vi "Over Awesome stuff.vi"() -> ()   [LabVIEW 2017]
uses:
  Gluing Procedure.lvclass
panel:
  out "Gluing Procedure out":refnum<class "Gluing Procedure.lvclass">
  in  "Gluing Procedure in":refnum<class "Gluing Procedure.lvclass">
  out "error out":errorcluster
  in  "error in":errorcluster
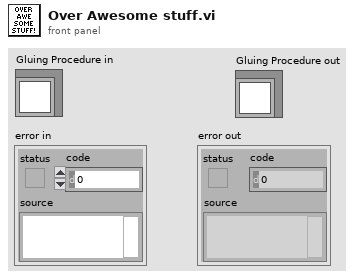
[diagram p1: front panel]
types:
  T1 = typedef "Configure.ctl" = cluster{"Has been run?":bool, "Active Paths":T2, "Glue Pathways":T3, "Chuck Module Used for BBM:":T5}
  T2 = typedef "Active Paths.ctl" = bool[]
  T3 = typedef "Glue Paths.ctl" = T4[]
  T4 = typedef "Glue Path.ctl" = cluster{"HDI Slot ":i32, "Stamp Slot":i32, "Glue Slot":i32, "Weight Slot":i32, "BBM Slot":i32}
  T5 = typedef "BBM Chuck Used.ctl" = i32
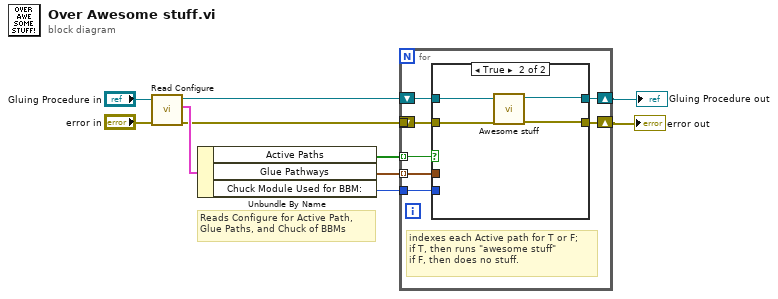
[diagram p0: block diagram]
diagram:
  # "Reads Configure for Active Path, \nGlue Paths, and Chuck of BBMs"
  n1 = call "Read Configure.vi"("error in (no error)"="error in", "Gluing Procedure in"="Gluing Procedure in") -> ("error out"=w1:errorcluster, "Configure"=w6:T1, "Gluing Procedure out"=w2:refnum<class "Gluing Procedure.lvclass">)  [unwired: 7 in]
  n2 = Unbundle By Name(w6) -> ("Active Paths"=w5:T2, "Glue Pathways"=w4:T3, "Chuck Module Used for BBM:"=w3:T5)
  n3 = for {
    tunnel: w5 -> [w17] mode=indexing
    tunnel: w4 -> [w16] mode=indexing
    shift-right: [w14] -> w8
    shift-left: w2 -> [w15]
    tunnel: w3 -> [w13]
    tunnel: w1 -> [w12]
    shift-right: [w11] -> w7
    shift-left: _ -> [_]
    # "indexes each Active path for T or F; \nif T, then runs \"awesome stuff\"\nif F, then does no stuff."
    n4 = case shown="True" w17 {
      tunnel: w16 -> [_ _]
      tunnel: w15 -> [w19 w23]
      tunnel: [w19 w21] -> w14
      tunnel: w13 -> [_ _]
      tunnel: w12 -> [w18 w22]
      tunnel: [w18 w20] -> w11
      frame False {
      }
      frame True {
        n5 = call "Awesome stuff.vi"("error in"=w22, "Gluing Procedure in"=w23) -> ("error out"=w20:errorcluster, "Gluing Procedure out"=w21:refnum<class "Gluing Procedure.lvclass">)  [unwired: 8 in]
      }
    }
  }
  "error out" <- w7
  "Gluing Procedure out" <- w8
